vi "ReadTempAndUpdateFPGA.vi"(8 "error in (no error)":errorcluster, 10 "TempThreshold":dbl=150.0, 11 "FPGA VI Reference":T1) -> (0 "error out":errorcluster)   [LabVIEW 2024]
uses:
  FPGA VI Ref.ctl
  <vilib>/Utility/error.llb/Error Cluster From Error Code.vi
  <vilib>/rvi/errors/niLvFpgaAdjustHostInterfaceError.vi
  <vilib>/rvi/interface/nirviReadWriteControl/nirviReadWriteControl.xnode
  <vilib>/rvi/interface/Simulation/niFpgaSimulationCallBeginRW.vi
  NiFpgaLv.dll
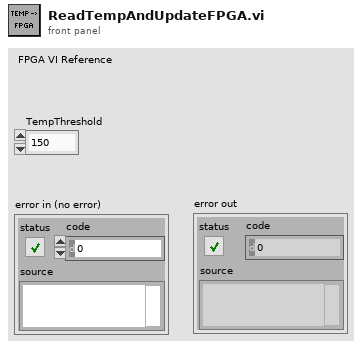
[diagram p1: front panel]
types:
  T1 = typedef "FPGA VI Ref.ctl" = refnum<k20>
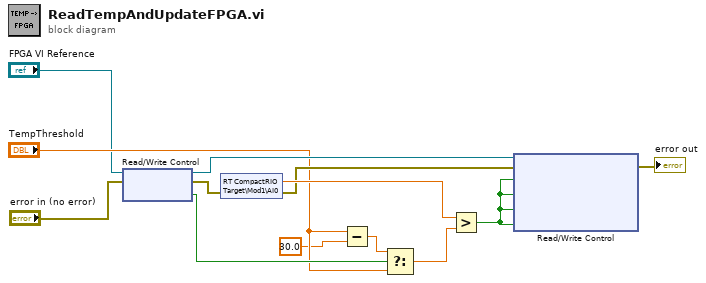
[diagram p0: block diagram]
diagram:
  n1 = xnode "Read/Write Control"("FPGA VI Reference In"="FPGA VI Reference", "error in"="error in (no error)") -> ("FPGA VI Reference Out"=w8:T1, "error out"=w9:errorcluster, "Löyly LED"=w6:bool)
  n2 = shared-variable "RT CompactRIO Target\\Mod1\\AI0"(error in=w9) -> (w12:dbl, error out=w7:errorcluster)
  n3 = Subtract(x="TempThreshold", y=30.0) -> (x-y=w4:dbl)
  n4 = Select(t=w4, s=w6, f="TempThreshold") -> (s? t:f=w5:dbl)
  n5 = Greater?(x=w12, y=w5) -> (0:w11:bool)
  n6 = xnode "Read/Write Control"("FPGA VI Reference In"=w8, "error in"=w7, "Aromi Pump Enable"=w11, "Löyly Valve Enable"=w11, "Aromi LED"=w11, "Löyly LED"=w11) -> ("error out"=→"error out":errorcluster)  [unwired: 1 out]
